vi "FilterFile.vi"(8 "FileType":string(combo)="WL", 10 "Path":path, 11 "Filenames":string[](array[string])) -> (0 "RW_Up":T1, 1 "FW_Up":T1, 2 "RW_Down":T1, 3 "FW_Down":T1, 4 "FileOK":bool, 5 "Array Out":string[](array[string]))   [LabVIEW 2017]
uses:
  <vilib>/Utility/file.llb/Read Delimited Spreadsheet (DBL).vi
panel:
  out "substring":string
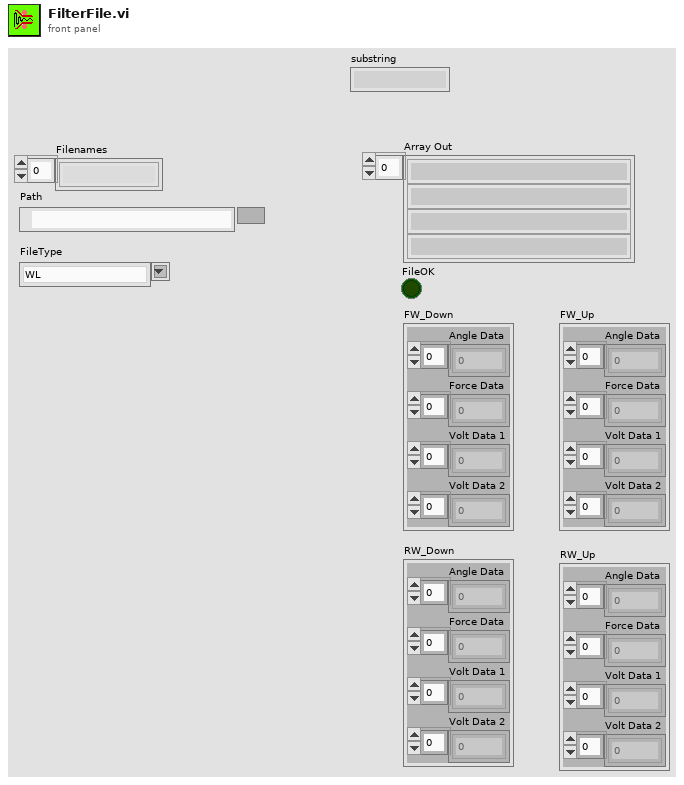
[diagram p1: front panel]
types:
  T1 = cluster{"Angle Data":dbl[], "Force Data":dbl[], "Volt Data 1":dbl[], "Volt Data 2":dbl[]}
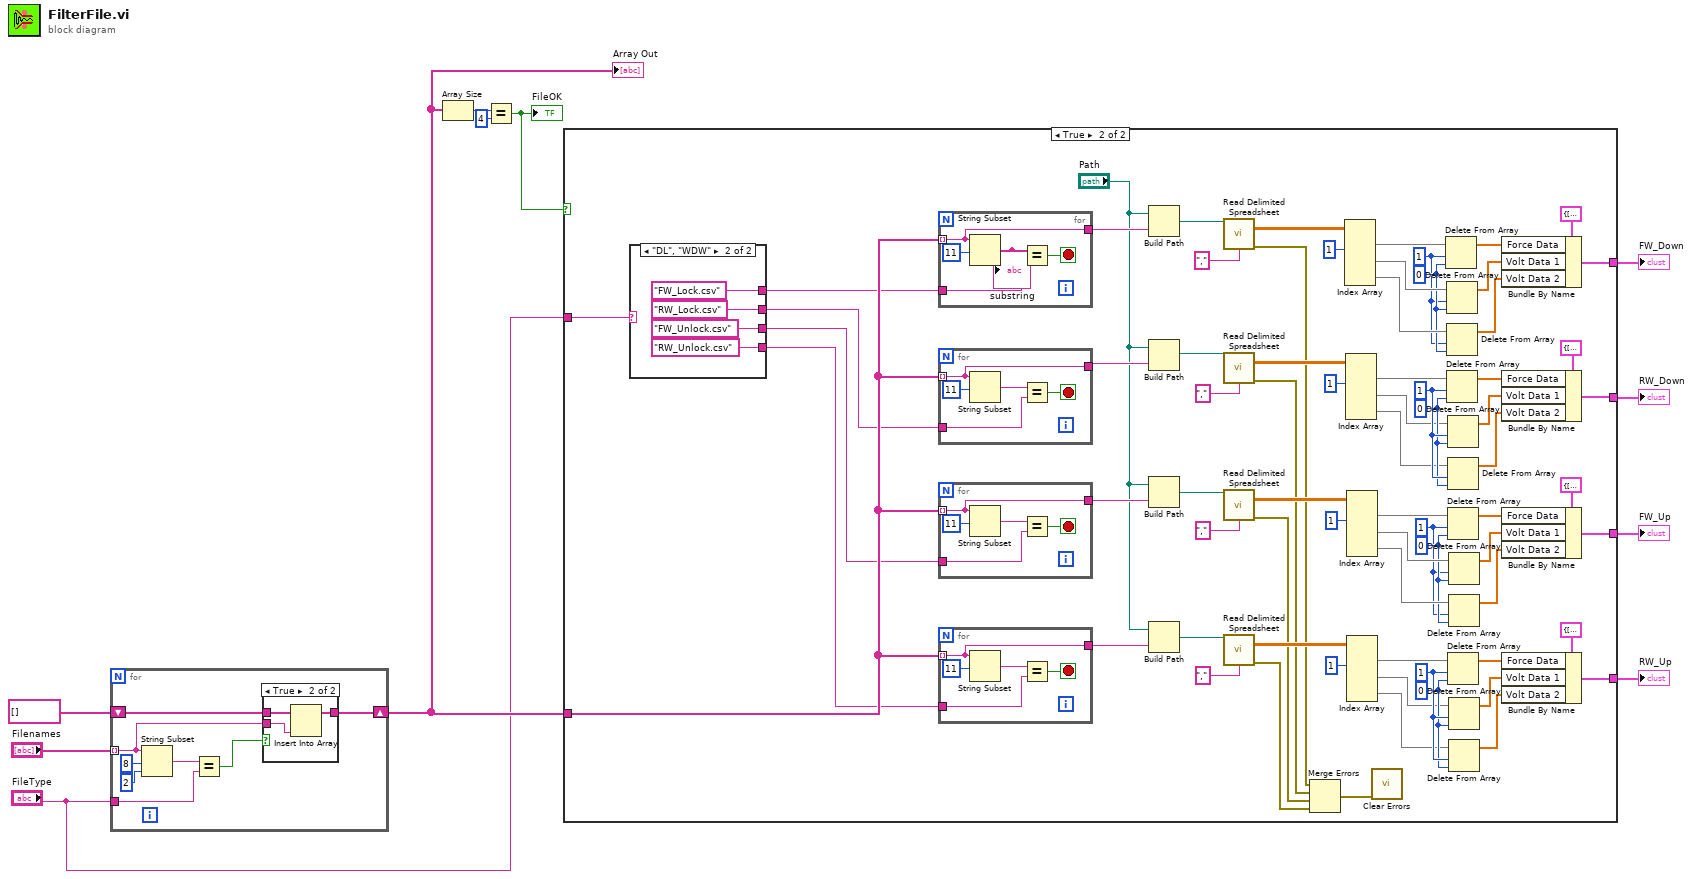
[diagram p0: block diagram]
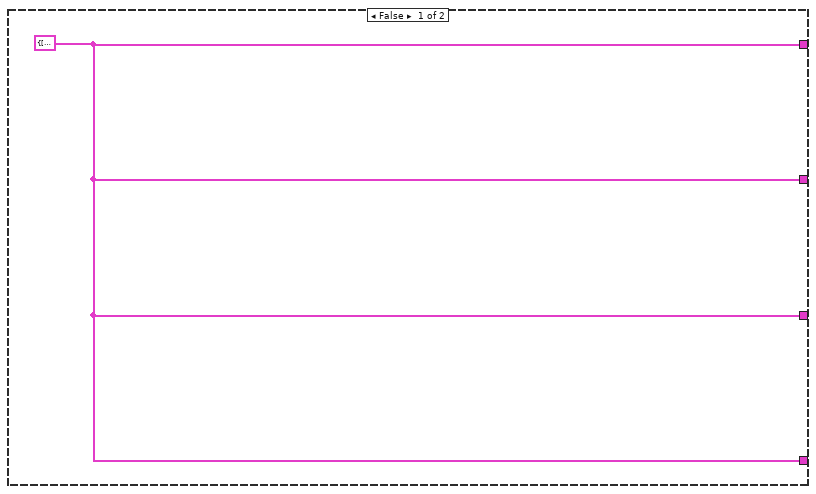
[diagram p2: hidden frame]
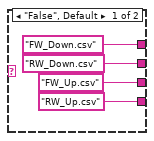
[diagram p3: hidden frame]
diagram:
  n1 = for {
    tunnel: "Filenames" -> [w14] mode=indexing
    tunnel: "FileType" -> [w16]
    shift-right: [w12] -> w2
    shift-left: string[] [] ("WL_Array") -> [w13]
    n2 = String Subset(string=w14, offset (0)=8, length (rest)=2 ("length (rest)")) -> (substring=w17:string)
    n3 = Equal?(x=w17, y=w16) -> (x = y?=w15:bool)
    n4 = case shown="True" w15 {
      tunnel: w14 -> [_ w23]
      tunnel: w13 -> [w20 w22]
      tunnel: [w20 w21] -> w12
      frame False {
      }
      frame True {
        n5 = Insert Into Array(array=w22, new element=w23) -> (w21:string[])  [unwired: 1 in]
      }
    }
  }
  "Array Out" <- w2
  n6 = Array Size(array=w2) -> (size(s)=w10:i32)
  n7 = Equal?(x=w10, y=4) -> (x = y?=w8:bool)
  "FileOK" <- w8
  n8 = case shown="True" w8 {
    tunnel: w2 -> [_ w83]
    tunnel: [w24 w35] -> w7
    tunnel: [w24 w60] -> w6
    tunnel: [w24 w48] -> w5
    tunnel: [w24 w36] -> w4
    tunnel: "FileType" -> [_ w29]
    frame False {
      w24 = T1 {"Angle Data"=[], "Force Data"=[], "Volt Data 1"=[], "Volt Data 2"=[]} ("Analog FW Out")
    }
    frame True {
      w45 = 0 ("index")
      w46 = 1 ("length")
      w52 = 0 ("index")
      w51 = 1 ("length")
      w70 = 0 ("index")
      w71 = 1 ("length")
      w73 = 0 ("index")
      w72 = 1 ("length")
      n9 = case shown="\"DL\", \"WDW\"" w29 {
        tunnel: ["FW_Down.csv" ("FileType") "FW_Lock.csv" ("FileType")] -> w28
        tunnel: ["RW_Down.csv" ("FileType") "RW_Lock.csv" ("FileType")] -> w27
        tunnel: ["FW_Up.csv" ("FileType") "FW_Unlock.csv" ("FileType")] -> w26
        tunnel: ["RW_Up.csv" ("FileType") "RW_Unlock.csv" ("FileType")] -> w25
        frame "False", Default {
        }
        frame "DL", "WDW" {
        }
      }
      n10 = for {
        tunnel: w83 -> [w120] mode=indexing
        tunnel: w28 -> [w123]
        tunnel: [w120] -> w96
        stop <- w122 stop-if-true
        n11 = String Subset(string=w120, offset (0)=11) -> (substring=w121:string)  [unwired: 1 in]
        "substring" <- w121
        n12 = Equal?(x=w121, y=w123) -> (x = y?=w122:bool)
      }
      n13 = for {
        tunnel: w83 -> [w115] mode=indexing
        tunnel: w27 -> [w118]
        tunnel: [w115] -> w95
        stop <- w117 stop-if-true
        n14 = String Subset(string=w115, offset (0)=11) -> (substring=w116:string)  [unwired: 1 in]
        n15 = Equal?(x=w116, y=w118) -> (x = y?=w117:bool)
      }
      n16 = for {
        tunnel: w83 -> [w110] mode=indexing
        tunnel: w26 -> [w113]
        tunnel: [w110] -> w94
        stop <- w112 stop-if-true
        n17 = String Subset(string=w110, offset (0)=11) -> (substring=w111:string)  [unwired: 1 in]
        n18 = Equal?(x=w111, y=w113) -> (x = y?=w112:bool)
      }
      n19 = for {
        tunnel: w83 -> [w105] mode=indexing
        tunnel: w25 -> [w108]
        tunnel: [w105] -> w93
        stop <- w107 stop-if-true
        n20 = String Subset(string=w105, offset (0)=11) -> (substring=w106:string)  [unwired: 1 in]
        n21 = Equal?(x=w106, y=w108) -> (x = y?=w107:bool)
      }
      n22 = Build Path(base path="Path", name or relative path=w96) -> (appended path=w91:path)
      n23 = Build Path(base path="Path", name or relative path=w95) -> (appended path=w86:path)
      n24 = Build Path(base path="Path", name or relative path=w94) -> (appended path=w85:path)
      n25 = Build Path(base path="Path", name or relative path=w93) -> (appended path=w84:path)
      n26 = call-poly <vilib>:"Read Delimited Spreadsheet.vi"("file path (dialog if empty)"=w91, "delimiter (\\t)"="," ("delimiter (\\t)")) -> ("all rows"=w75:dbl[][], "error out"=w34:errorcluster)  [unwired: 8 in, 4 out]
      n27 = call-poly <vilib>:"Read Delimited Spreadsheet.vi"("file path (dialog if empty)"=w86, "delimiter (\\t)"="," ("delimiter (\\t)")) -> ("all rows"=w61:dbl[][], "error out"=w33:errorcluster)  [unwired: 8 in, 4 out]
      n28 = call-poly <vilib>:"Read Delimited Spreadsheet.vi"("file path (dialog if empty)"=w85, "delimiter (\\t)"="," ("delimiter (\\t)")) -> ("all rows"=w50:dbl[][], "error out"=w32:errorcluster)  [unwired: 8 in, 4 out]
      n29 = call-poly <vilib>:"Read Delimited Spreadsheet.vi"("file path (dialog if empty)"=w84, "delimiter (\\t)"="," ("delimiter (\\t)")) -> ("all rows"=w37:dbl[][], "error out"=w31:errorcluster)  [unwired: 8 in, 4 out]
      n30 = Merge Errors(w34, w33, w32, w31) -> (w30:errorcluster)
      n31 = Index Array(array=w75, index (col) #1=1 ("disabled index (col)")) -> (element #1=w77:dbl[], element #2=w79:dbl[], element #3=w80:dbl[])  [unwired: 5 in]
      n32 = Index Array(array=w61, index (col) #1=1 ("disabled index (col)")) -> (element #1=w67:dbl[], element #2=w65:dbl[], element #3=w64:dbl[])  [unwired: 5 in]
      n33 = Index Array(array=w50, index (col) #1=1 ("disabled index (col)")) -> (element #1=w54:dbl[], element #2=w56:dbl[], element #3=w57:dbl[])  [unwired: 5 in]
      n34 = Index Array(array=w37, index (col) #1=1 ("disabled index (col)")) -> (element #1=w43:dbl[], element #2=w41:dbl[], element #3=w40:dbl[])  [unwired: 5 in]
      n35 = call <vilib>:"Clear Errors.vi"("error in (no error)"=w30) -> ()  [unwired: 5 in, 2 out]
      n36 = Delete From Array(array=w77, length=w72, index=w73) -> (array with subset deleted=w78:dbl[])  [unwired: 1 out]
      n37 = Delete From Array(array=w79, length=w72, index=w73) -> (array with subset deleted=w81:dbl[])  [unwired: 1 out]
      n38 = Delete From Array(array=w80, length=w72, index=w73) -> (array with subset deleted=w82:dbl[])  [unwired: 1 out]
      n39 = Delete From Array(array=w67, length=w71, index=w70) -> (array with subset deleted=w66:dbl[])  [unwired: 1 out]
      n40 = Delete From Array(array=w65, length=w71, index=w70) -> (array with subset deleted=w63:dbl[])  [unwired: 1 out]
      n41 = Delete From Array(array=w64, length=w71, index=w70) -> (array with subset deleted=w62:dbl[])  [unwired: 1 out]
      n42 = Delete From Array(array=w54, length=w51, index=w52) -> (array with subset deleted=w55:dbl[])  [unwired: 1 out]
      n43 = Delete From Array(array=w43, length=w46, index=w45) -> (array with subset deleted=w42:dbl[])  [unwired: 1 out]
      n44 = Delete From Array(array=w56, length=w51, index=w52) -> (array with subset deleted=w58:dbl[])  [unwired: 1 out]
      n45 = Delete From Array(array=w57, length=w51, index=w52) -> (array with subset deleted=w59:dbl[])  [unwired: 1 out]
      n46 = Delete From Array(array=w41, length=w46, index=w45) -> (array with subset deleted=w39:dbl[])  [unwired: 1 out]
      n47 = Delete From Array(array=w40, length=w46, index=w45) -> (array with subset deleted=w38:dbl[])  [unwired: 1 out]
      n48 = Bundle By Name(cluster=T1 {"Angle Data"=[], "Force Data"=[], "Volt Data 1"=[], "Volt Data 2"=[]} ("Analog FW Out"), "Force Data"=w78, "Volt Data 1"=w81, "Volt Data 2"=w82) -> (w35:T1)
      n49 = Bundle By Name(cluster=T1 {"Angle Data"=[], "Force Data"=[], "Volt Data 1"=[], "Volt Data 2"=[]} ("Analog FW Out"), "Force Data"=w66, "Volt Data 1"=w63, "Volt Data 2"=w62) -> (w60:T1)
      n50 = Bundle By Name(cluster=T1 {"Angle Data"=[], "Force Data"=[], "Volt Data 1"=[], "Volt Data 2"=[]} ("Analog FW Out"), "Force Data"=w55, "Volt Data 1"=w58, "Volt Data 2"=w59) -> (w48:T1)
      n51 = Bundle By Name(cluster=T1 {"Angle Data"=[], "Force Data"=[], "Volt Data 1"=[], "Volt Data 2"=[]} ("Analog FW Out"), "Force Data"=w42, "Volt Data 1"=w39, "Volt Data 2"=w38) -> (w36:T1)
    }
  }
  "FW_Down" <- w7
  "RW_Down" <- w6
  "FW_Up" <- w5
  "RW_Up" <- w4
